vi "AffinityPropagation.vi"(8 "error in":errorcluster) -> (0 "error out":errorcluster, 3 "out":refnum<class "AffinityPropagation.lvclass">)   [LabVIEW 2020]
doc: "Perform Affinity Propagation Clustering of data.\n\n Read more in the :ref:`User Guide <affinity_propagation>`.\n\n Parameters\n ----------\n damping : float, default=0.5\n Damping factor (between 0.5 and 1) is the extent to\n which the current value is maintained relative to\n incoming values (weighted 1 - damping). This in order\n to avoid numerical oscillations when updating these\n values (messages).\n\n max_iter : int, default=200\n Maximum number of iterations.\n\n convergence_iter : int, default=15\n Number of iterations with no change in the number\n of estimated clusters that stops the convergence.\n\n copy : bool, default=True\n Make a copy of input data.\n\n preference : array-like of shape (n_samples,) or float, default=None\n Preferences for each point - points with larger values of\n preferences are more likely to be chosen as exemplars. The number\n of exemplars, ie of clusters, is influenced by the input\n preferences value. If the preferences are not passed as arguments,\n they will be set to the median of the input similarities.\n\n affinity : {'euclidean', 'precomputed'}, default='euclidean'\n Which affinity to use. At the moment 'precomputed' and\n ``euclidean`` are supported. 'euclidean' uses the\n negative squared euclidean distance between points.\n\n verbose : bool, default=False\n Whether to be verbose.\n\n random_state : int, RandomState instance or None, default=0\n Pseudo-random number generator to control the starting state.\n Use an int for reproducible results across function calls.\n See the :term:`Glossary <random_state>`.\n\n .. versionadded:: 0.23\n this parameter was previously hardcoded as 0.\n\n Attributes\n ----------\n cluster_centers_indices_ : ndarray of shape (n_clusters,)\n Indices of cluster centers.\n\n cluster_centers_ : ndarray of shape (n_clusters, n_features)\n Cluster centers (if affinity != ``precomputed``).\n\n labels_ : ndarray of shape (n_samples,)\n Labels of each point.\n\n affinity_matrix_ : ndarray of shape (n_samples, n_samples)\n Stores the affinity matrix used in ``fit``.\n\n n_iter_ : int\n Number of iterations taken to converge.\n\n Notes\n -----\n For an example, see :ref:`examples/cluster/plot_affinity_propagation.py\n <sphx_glr_auto_examples_cluster_plot_affinity_propagation.py>`.\n\n The algorithmic complexity of affinity propagation is quadratic\n in the number of points.\n\n When ``fit`` does not converge, ``cluster_centers_`` becomes an empty\n array and all training samples will be labelled as ``-1``. In addition,\n ``predict`` will then label every sample as ``-1``.\n\n When all training samples have equal similarities and equal preferences,\n the assignment of cluster centers and labels depends on the preference.\n If the preference is smaller than the similarities, ``fit`` will result in\n a single cluster center and label ``0`` for every sample. Otherwise, every\n training sample becomes its own cluster center and is assigned a unique\n label.\n\n References\n ----------\n\n Brendan J. Frey and Delbert Dueck, \"Clustering by Passing Messages\n Between Data Points\", Science Feb. 2007\n\n \nAvailable methods:\nGet Attributes\nGet Params\nSet Params"
uses:
  AffinityPropagation.lvclass
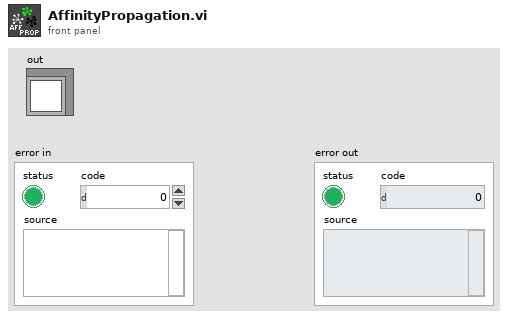
[diagram p1: front panel]
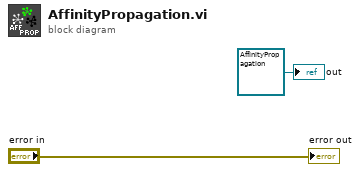
[diagram p0: block diagram]
diagram:
  "out" <- refnum<class "AffinityPropagation.lvclass"> refnum ("model")
  "error out" <- "error in"
